vi "MagnetoGUI.vi"() -> ()   [LabVIEW 2016]
uses:
  controls/GUI Parameter.ctl
  controls/State.ctl
  controls/Data.ctl
panel:
  out "Tab Control":T1(tab)
  out "Aktueller Zustand":string
  in  "Taster Einstellungen":bool
  in  "Anz. Messpunkte Kommutierungskurve":i8=16 caption="Anz. Messpunkte\nKommutierungskurve" min=10 max=30 step=1
  out "Hystereseschleife und Kom.Kurve / Preview":cluster{dbl[], dbl[]}[](graph) caption="XY Graph"
  in  "Plot_Speichern":bool
  out "Status":bool
  in  "Start Button":bool
  in  "Maximieren":bool
  in  "GUI Parameter":T2={"Eisenquerschnitt [mm^2]"=30.0, "Wirksame Länge [cm]"=94.0, "Primärwindungszahl"=700.0, "Sekundärwindungszahl"=700.0, "Messwiderstand [Ohm]"=1.0, "Spannungsteilerverhaeltnis (1/x)"=1.0, "Probenbezeichnung"="", "Dichte des Eisens [g/cm^3]"=7.84, "magn. Flussdichte [T]"=2.0, "Frequenz [Hz]"=50.0, "Namen"="", "Gruppe"=""} {"Frequenz [Hz]" min=15.0 max=15000.0; "magn. Flussdichte [T]" min=0.001 max=5.0 step=0.05; "Dichte des Eisens [g/cm^3]" min=1.0 max=50.0 step=0.01; "Spannungsteilerverhaeltnis (1/x)" step=0.05; "Sekundärwindungszahl" min=1.0 max=1500.0; "Primärwindungszahl" min=1.0 max=1500.0; "Wirksame Länge [cm]" min=1.0 max=1000.0; "Eisenquerschnitt [mm^2]" min=1.0 max=10000.0}
  in  "Kommutierungskurve messen?":bool caption="Kommutierungskurve\nMessen?"
  in  "Maximal zulässiger Strom [A]":dbl=3.0 min=0.0 max=5.0 step=0.05
  in  "Minimale Spannung [V]":dbl=0.02 min=0.0 max=10.0
  in  "Maximale Spannung [V]":dbl=10.0 min=0.0 max=10.0
  out "Faktor2":dbl
  out "Faktor1":dbl
  out "TP":dbl caption="Theoretische Primärwindungszahl"
  in  "Taster Hauptansicht":bool
  in  "VISA Name Oszilloscope":refnum<visa-resource-name>="USB0::0x0957::0x179B::MY54313507::INSTR"
  in  "VISA Name Frequenzgen.":refnum<visa-resource-name>="USB0::0x0957::0x0407::MY44043889::INSTR"
  in  "Anzahl der Oszi-Messpunkte":i32=2000 min=2000 max=2000 step=1
  out "Bmax [T]":dbl
  out "Hmax [A/m]":dbl
  out "Koerzitivfeldstärke [A/m]":dbl caption="Koerzitiv-\nfeldstärke [A/m]"
  out "Remanenz [T]":dbl
  in  "Excel Export":bool
  out "Gruppe":string
  out "Namen":string
  out "Frequenz [Hz]":dbl
  out "magn. Flussdichte [T]":dbl
  out "Dichte des Eisens [g/cm^3]":dbl
  out "Probenbezeichnung":string
  out "Spannungsteilerverhältnis (1/x)":dbl
  out "Messwiderstand [Ohm]":dbl
  out "Sekundärwindungszahl":dbl
  out "Primärwindungszahl":dbl
  out "Wirksame Länge [cm]":dbl
  out "Eisenquerschnitt [mm^2]":dbl
  in  "Minimieren":bool
  in  "Ansicht_Speichern":bool
  out "Hystereseschleife und Kom.Kurve":cluster{dbl[], dbl[]}[](graph) caption="XY Graph"
  in  "Plot_Speichern 2":bool
  out "Datum/Uhrzeit":timestamp format="%<%H:%M\n%d/%m/%y>T"
  out "Hystereseverluste [W]":dbl
  # "Meldung merkerstromüberwachung"
  # "Meldung Frequenzgen im Spannungslimit"
  # "Laborversuch: Magnetische Eigenschaften"
  # "Laborversuch: Magnetische Eigenschaften"
  # "Oszilloskop Messpunkte"
  # "System Setup"
  # "Frequenzgenerator"
  # "Strombegrenzung"
  # "Anzeige der berechneten Größen"
  # "Laborversuch: Magnetische Eigenschaften"
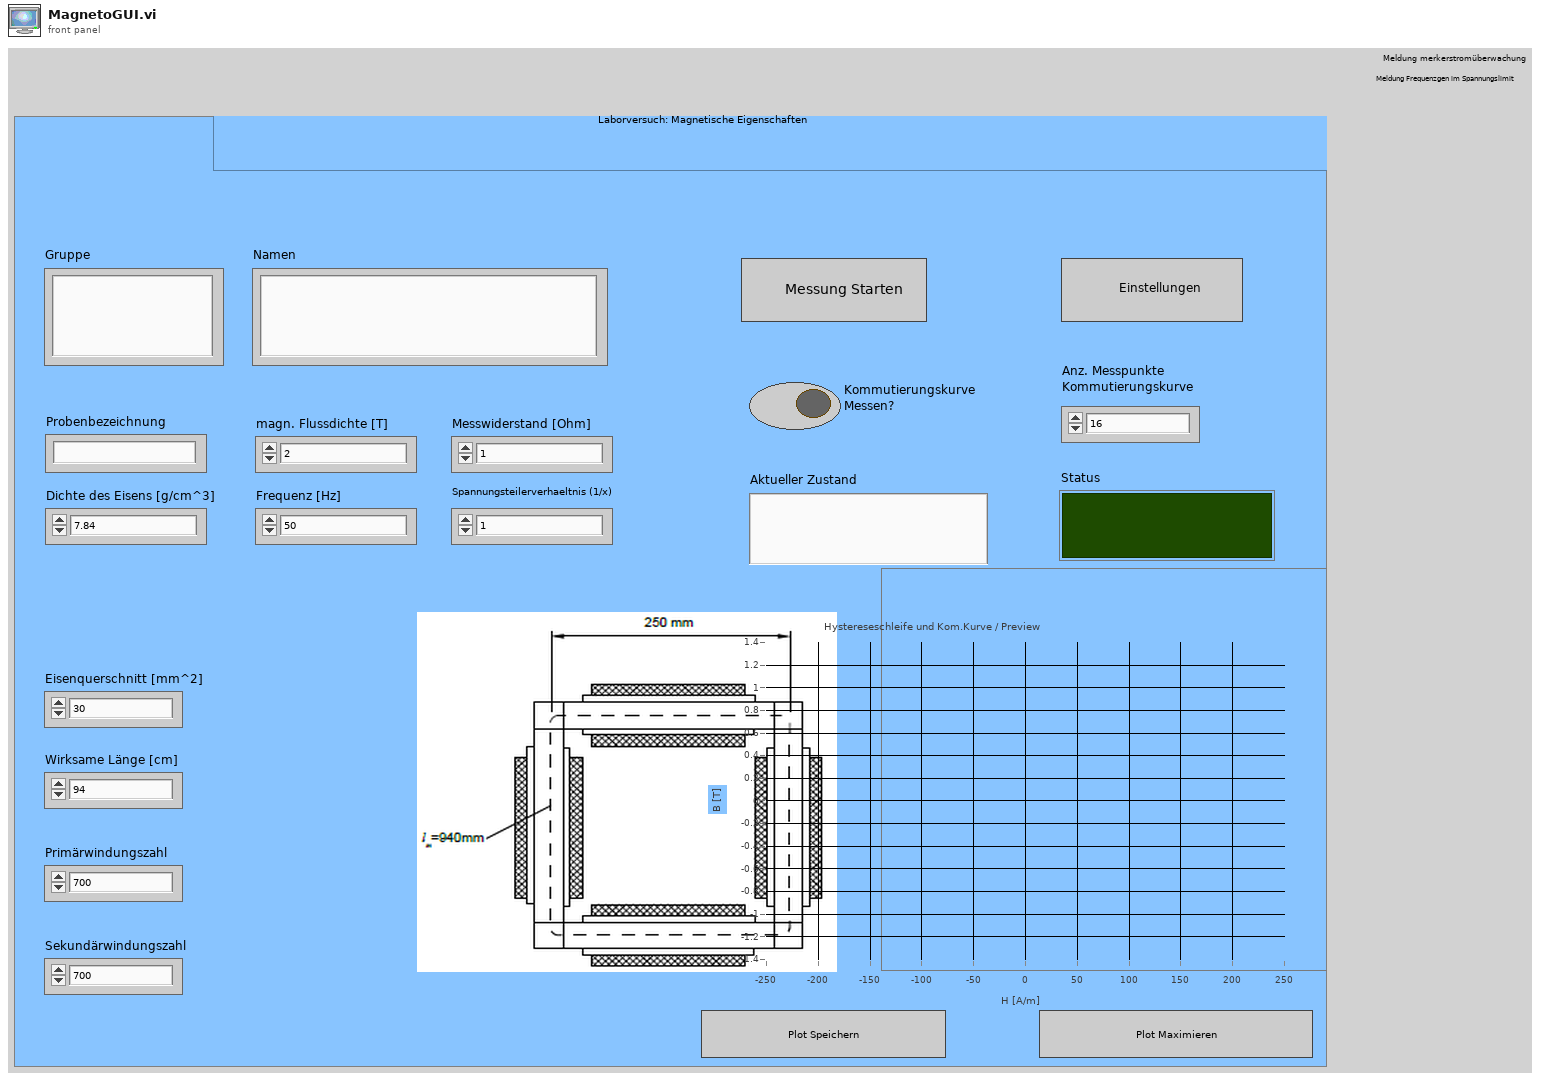
[diagram p1: front panel]
types:
  T1 = enum32{"Hauptansicht", "Optionen", "Plotansicht"}
  T2 = typedef "GUI Parameter.ctl" = cluster{"Eisenquerschnitt [mm^2]":dbl, "Wirksame Länge [cm]":dbl, "Primärwindungszahl":dbl, "Sekundärwindungszahl":dbl, "Messwiderstand [Ohm]":dbl, "Spannungsteilerverhaeltnis (1/x)":dbl, "Probenbezeichnung":string, "Dichte des Eisens [g/cm^3]":dbl, "magn. Flussdichte [T]":dbl, "Frequenz [Hz]":dbl, "Namen":string, "Gruppe":string}
  T3 = typedef "Data.ctl" = cluster{"GUI Einstellungen":cluster{"Maximale Spannung FG":dbl, "Faktor1":dbl, "Faktor2":dbl, "Theoretische Primärwindungszahl":dbl, "Anzahl der Messpunkte":i32, "VISA Name Oszilloscope":refnum<visa-resource-name>, "VISA Name Frequenzgenerator":refnum<visa-resource-name>, "Minimale Spannung FG":dbl, "Pfad für Messwerte und Plots":path, "Maximal Strom [A] ":dbl}, "GUI Daten":cluster{"Eisenquerschnitt [mm^2]":dbl, "Wirksame Länge [cm]":dbl, "Primärwindungszahl":dbl, "Sekundärwindungszahl":dbl, "Messwiderstand [Ohm]":dbl, "Spannungsteilerverhaeltnis (1/x)":dbl, "Probenbezeichnung":string, "Dichte des Eisens [g/cm^3]":dbl, "magn. Flussdichte [T]":dbl, "Frequenz [Hz]":dbl, "Namen":string, "Gruppe":string}, "Messung Hystereseschleife":cluster{"Hystereseverluste":dbl, "B - Hysterese Array":dbl[], "H - Hysterese Array":dbl[], "Hmax":dbl, "Bmax":dbl, "Remanenz":dbl, "Koerzitivfeldstärke":dbl}, "Messung Neukurve":cluster{"Neukurve Messen?":bool, "Anzahl Messpunkte Neukurve":i8, "B - Neukurve Array":dbl[], "H - Neukurve Array":dbl[]}, "Globale Variablen":cluster{"Max Spannung\nerreicht?":bool, "Min Spannung\nerreicht?":bool, "Keine Neu- oder\nKommutierungskurvenmessung\nmoeglich":bool, "bmax1":dbl, "bmin1":dbl, "bmax2":dbl, "bmin2":dbl, "Spannungsabweichung":dbl, "Tatsächliche Flussdichte":dbl, "Tatsächliche \nAnzahl Punkte":dbl, "hmax1":dbl, "hmin1":dbl, "hmax2":dbl, " Strombegrenzung aktiv?":bool, "Abbruch Messung":bool}}
  T4 = typedef "State.ctl" = enum16{"Initialisieren", "Warten auf Event", "Starten der Messung", "Initialisieren Hardware", "Flussdichte Einstellen", "Chk Flussdichte Anpassung", "Messung Hystereseschleife", "Entmagnetisieren", "Messung Kommutierungskurve", "Entmagnetisieren 2", "Ausgabe Diagramm", "Ende", "Plot aufnehmen", "Ansicht speichern", "Excel Export"}
  T5 = cluster{"Maximale Spannung FG":dbl, "Faktor1":dbl, "Faktor2":dbl, "Theoretische Primärwindungszahl":dbl, "Anzahl der Messpunkte":i32, "VISA Name Oszilloscope":refnum<visa-resource-name>, "VISA Name Frequenzgenerator":refnum<visa-resource-name>, "Minimale Spannung FG":dbl, "Pfad für Messwerte und Plots":path, "Maximal Strom [A] ":dbl}
  T6 = cluster{"Eisenquerschnitt [mm^2]":dbl, "Wirksame Länge [cm]":dbl, "Primärwindungszahl":dbl, "Sekundärwindungszahl":dbl, "Messwiderstand [Ohm]":dbl, "Spannungsteilerverhaeltnis (1/x)":dbl, "Probenbezeichnung":string, "Dichte des Eisens [g/cm^3]":dbl, "magn. Flussdichte [T]":dbl, "Frequenz [Hz]":dbl, "Namen":string, "Gruppe":string}
  T7 = cluster{"Max Spannung\nerreicht?":bool, "Min Spannung\nerreicht?":bool, "Keine Neu- oder\nKommutierungskurvenmessung\nmoeglich":bool, "bmax1":dbl, "bmin1":dbl, "bmax2":dbl, "bmin2":dbl, "Spannungsabweichung":dbl, "Tatsächliche Flussdichte":dbl, "Tatsächliche \nAnzahl Punkte":dbl, "hmax1":dbl, "hmin1":dbl, "hmax2":dbl, " Strombegrenzung aktiv?":bool, "Abbruch Messung":bool}
  T8 = cluster{"Max Spannung\nerreicht?":bool, "Min Spannung\nerreicht?":bool, "Keine Neu- oder\nKommutierungskurvenmessung\nmoeglich":bool, "bmax1":dbl, "bmin1":dbl, "bmax2":dbl, "bmin2":dbl, "Spannungsabweichung":dbl, "Tatsächliche Flussdichte":dbl, "Tatsächliche \nAnzahl Punkte":dbl, "hmax1":dbl, "hmin1":dbl, "hmax2":dbl, " Stromueberwachung aktiv?":bool, "Abbruch Messung":bool}
  T9 = cluster{"Hystereseverluste":dbl, "B - Hysterese Array":dbl[], "H - Hysterese Array":dbl[], "Hmax":dbl, "Bmax":dbl, "Remanenz":dbl, "Koerzitivfeldstärke":dbl}
  T10 = cluster{"H - Hysterese Array":dbl[], "B - Hysterese Array":dbl[]}
  T11 = cluster{"H - Neukurve Array":dbl[], "B - Neukurve Array":dbl[]}
  T12 = cluster{"H - Neukurve Array":dbl[], "B - Neukurve Array":dbl[]}[]
  T13 = typedef "imagedata.ctl" = cluster{"image type":i32, "image depth":i32, "image":u8[], "mask":u8[], "colors":u32[], "Rectangle":cluster{"left":i16, "top":i16, "right":i16, "bottom":i16}}
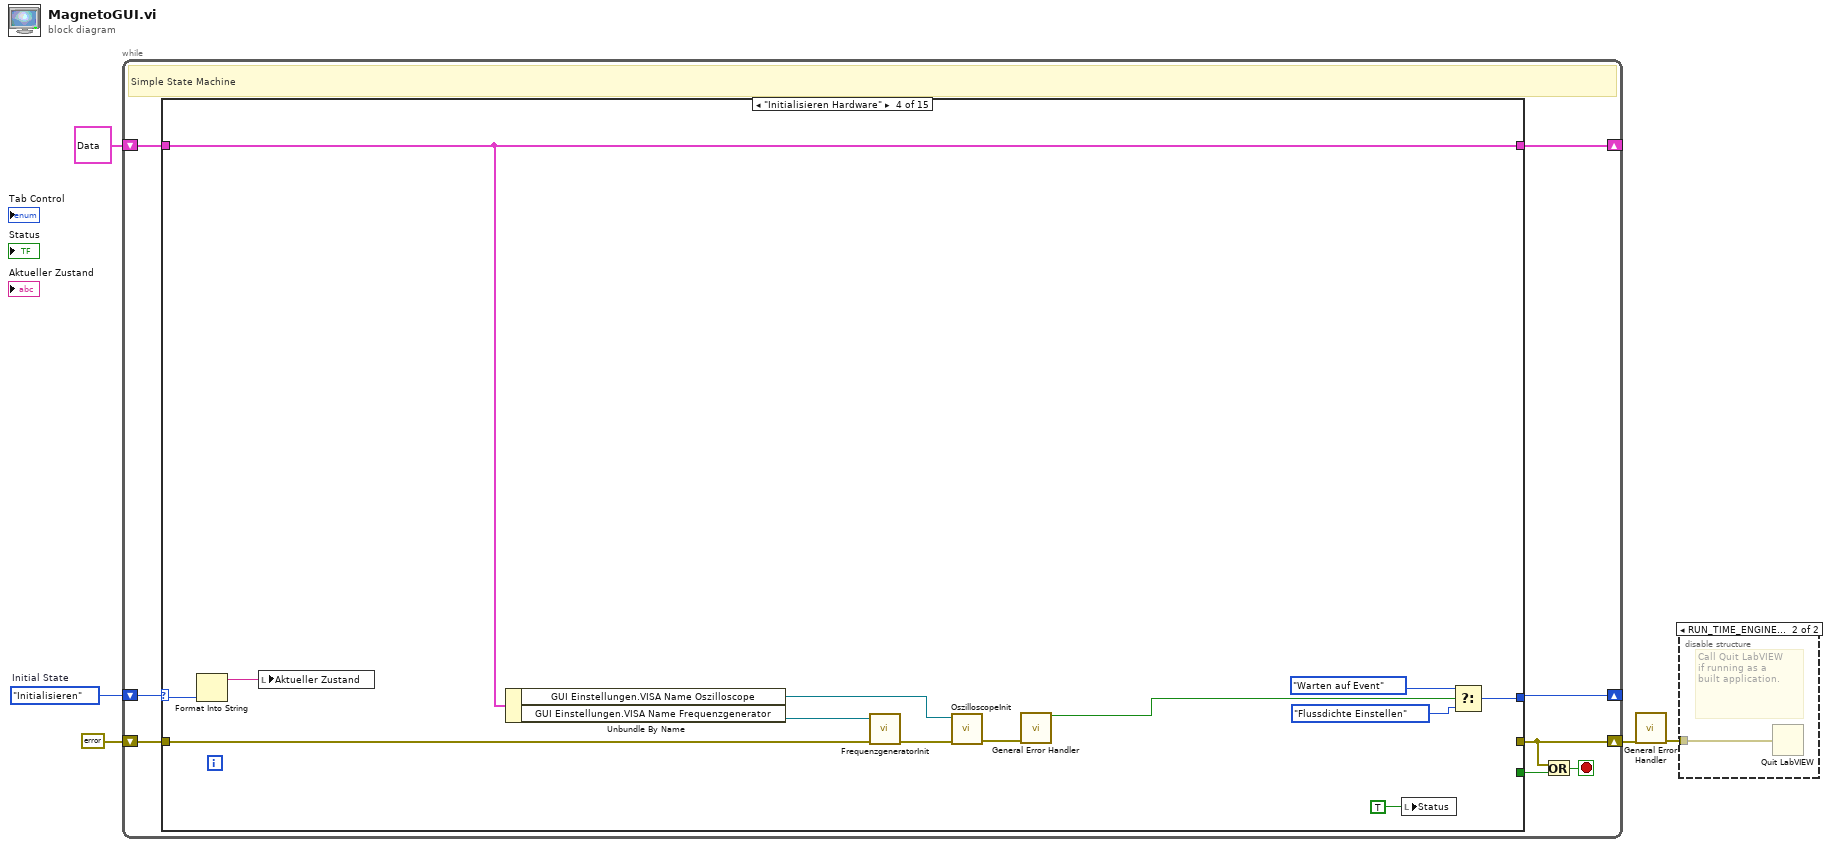
[diagram p0: block diagram]
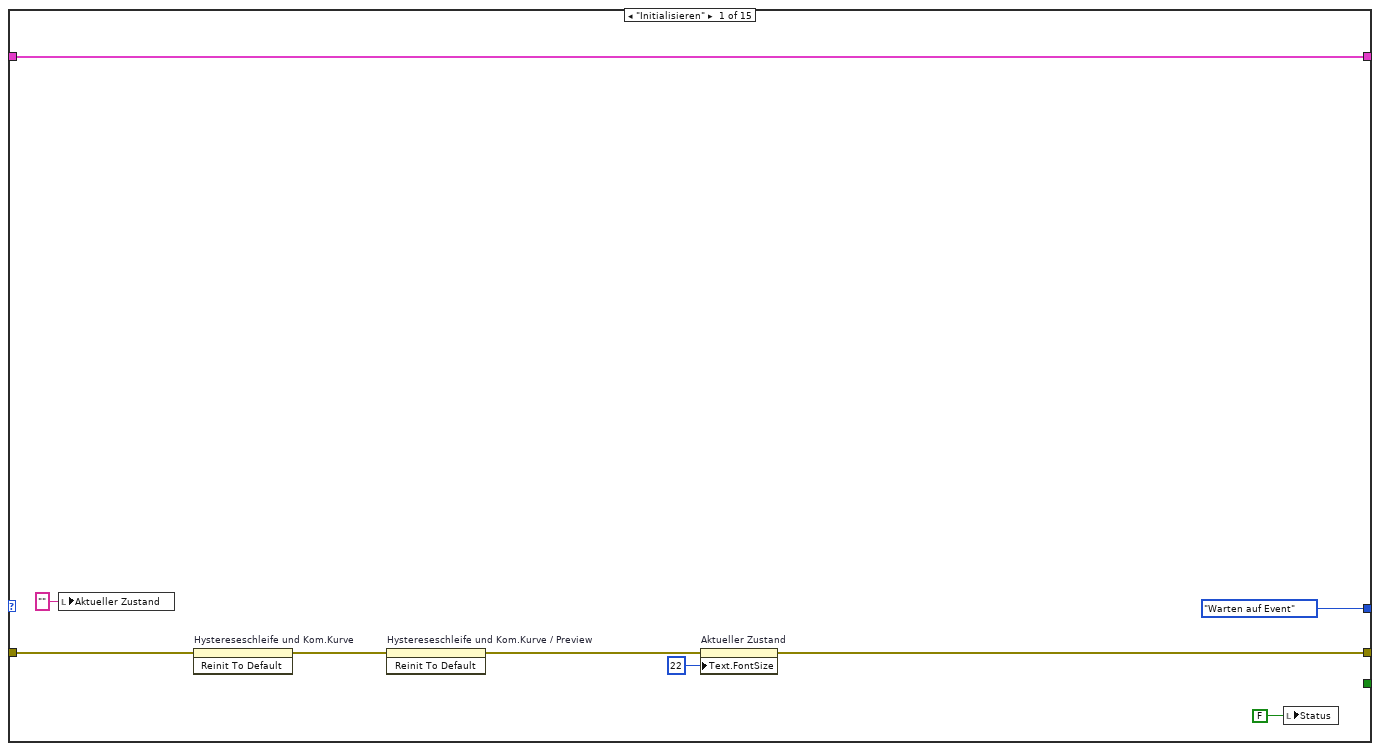
[diagram p3: hidden frame]
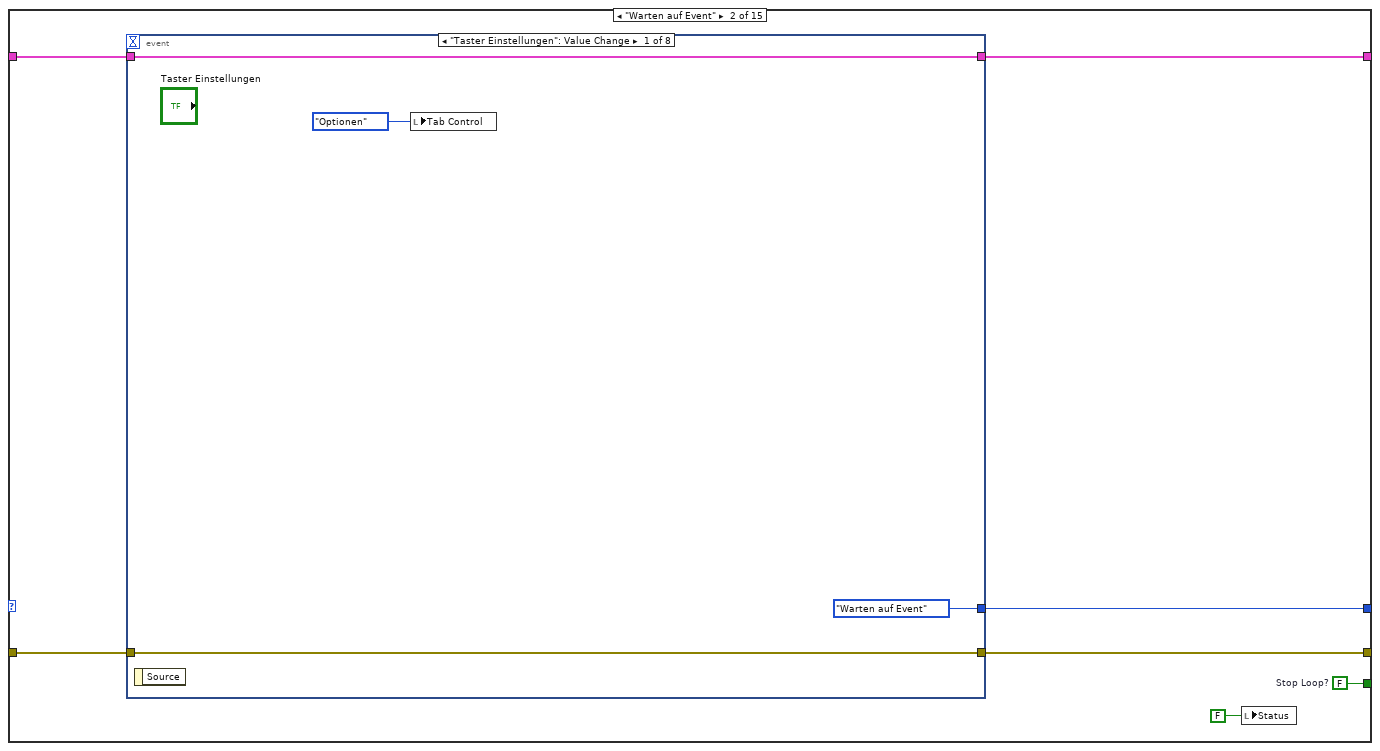
[diagram p4: hidden frame]
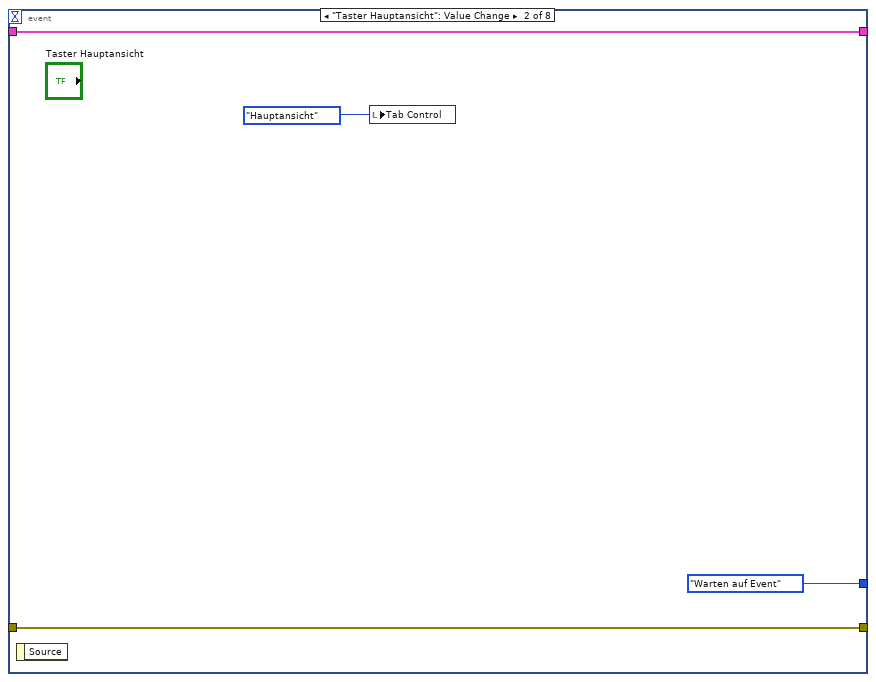
[diagram p5: hidden frame]
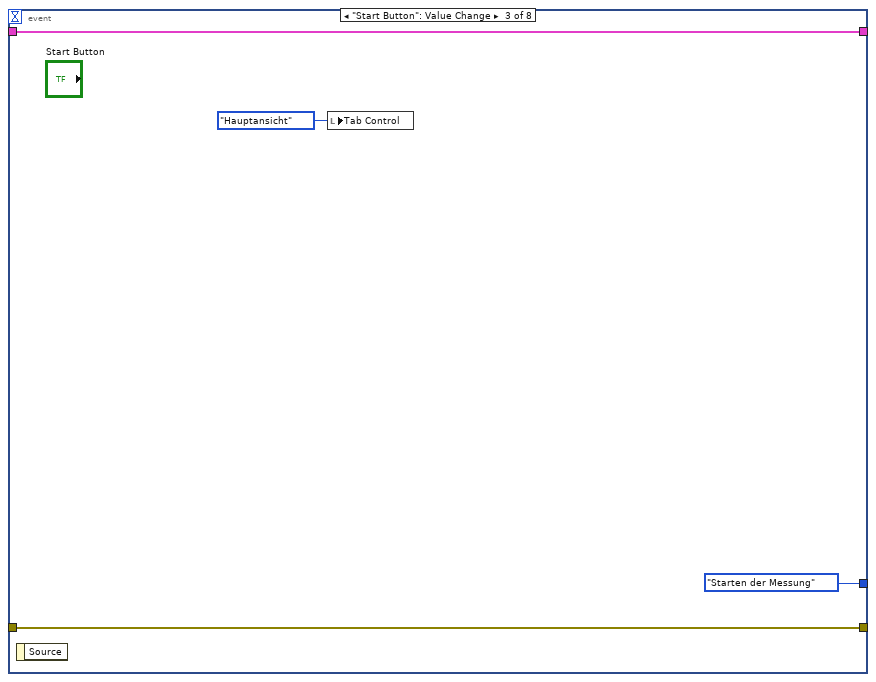
[diagram p6: hidden frame]
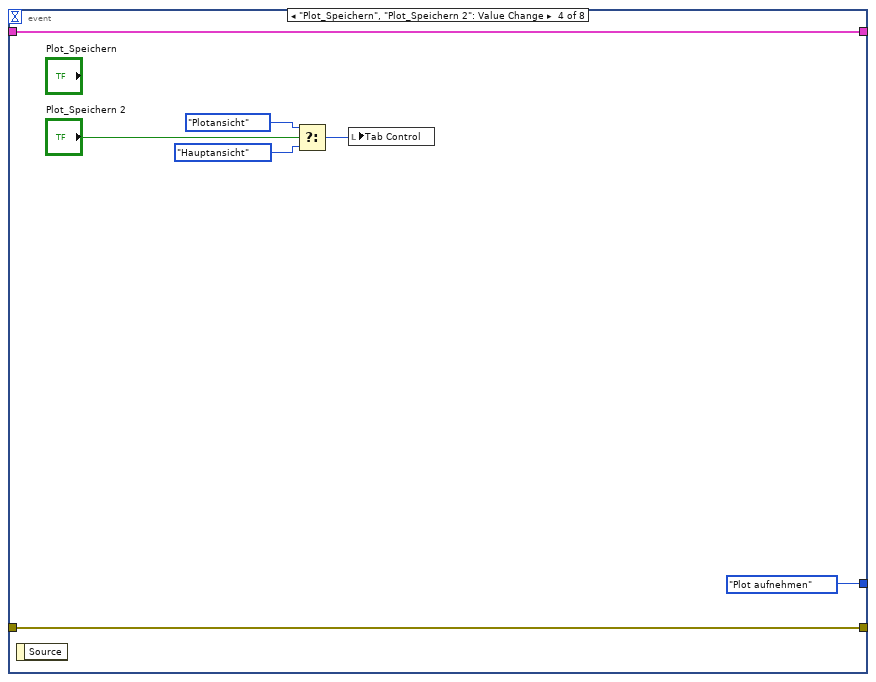
[diagram p7: hidden frame]
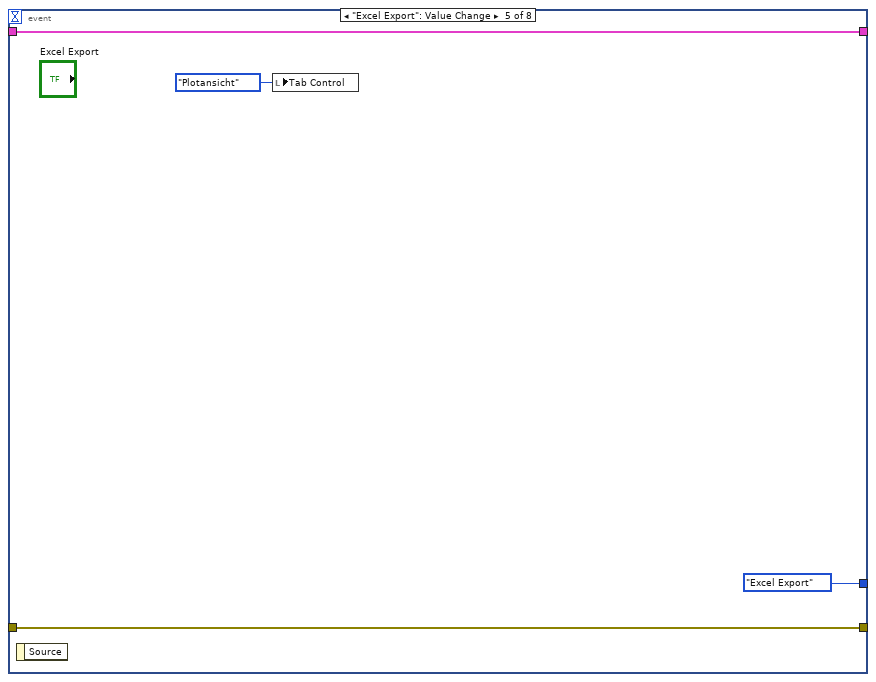
[diagram p8: hidden frame]
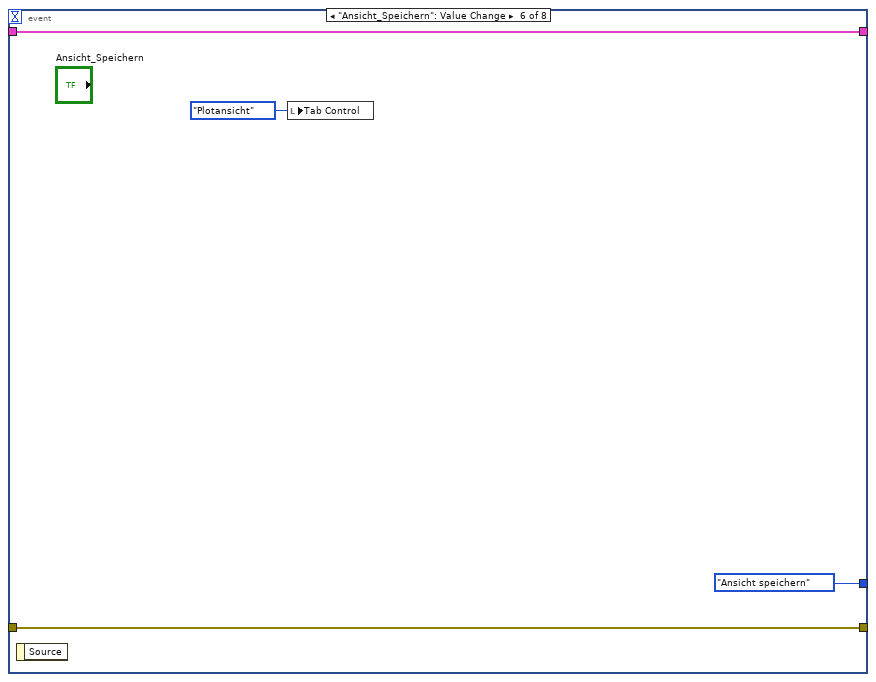
[diagram p9: hidden frame]
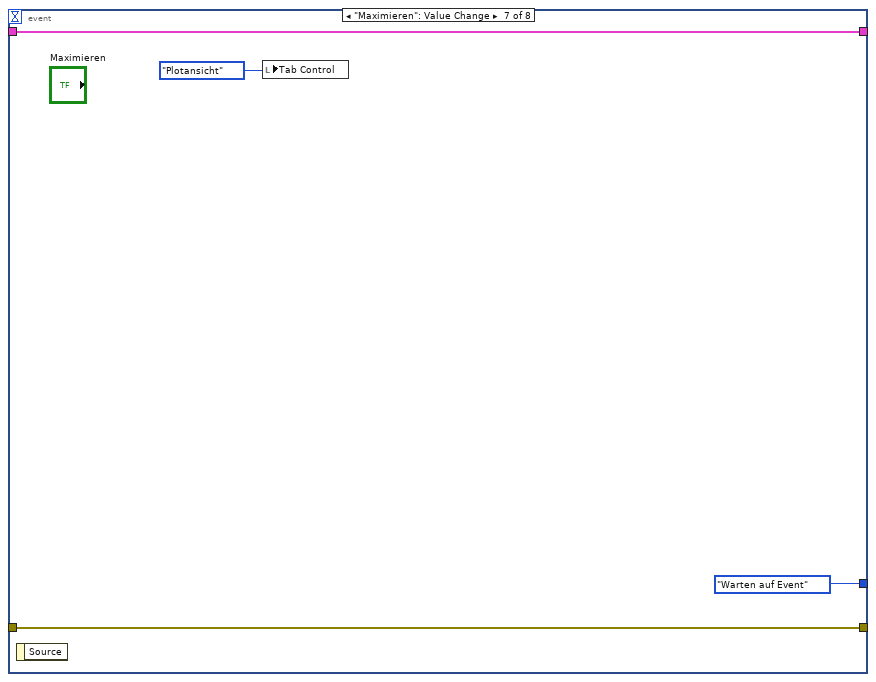
[diagram p10: hidden frame]
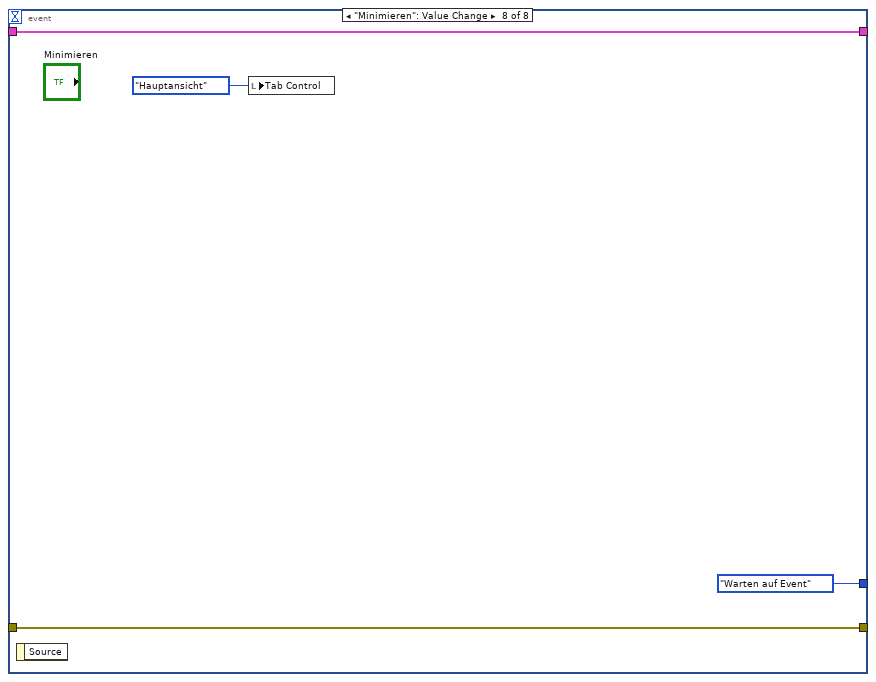
[diagram p11: hidden frame]
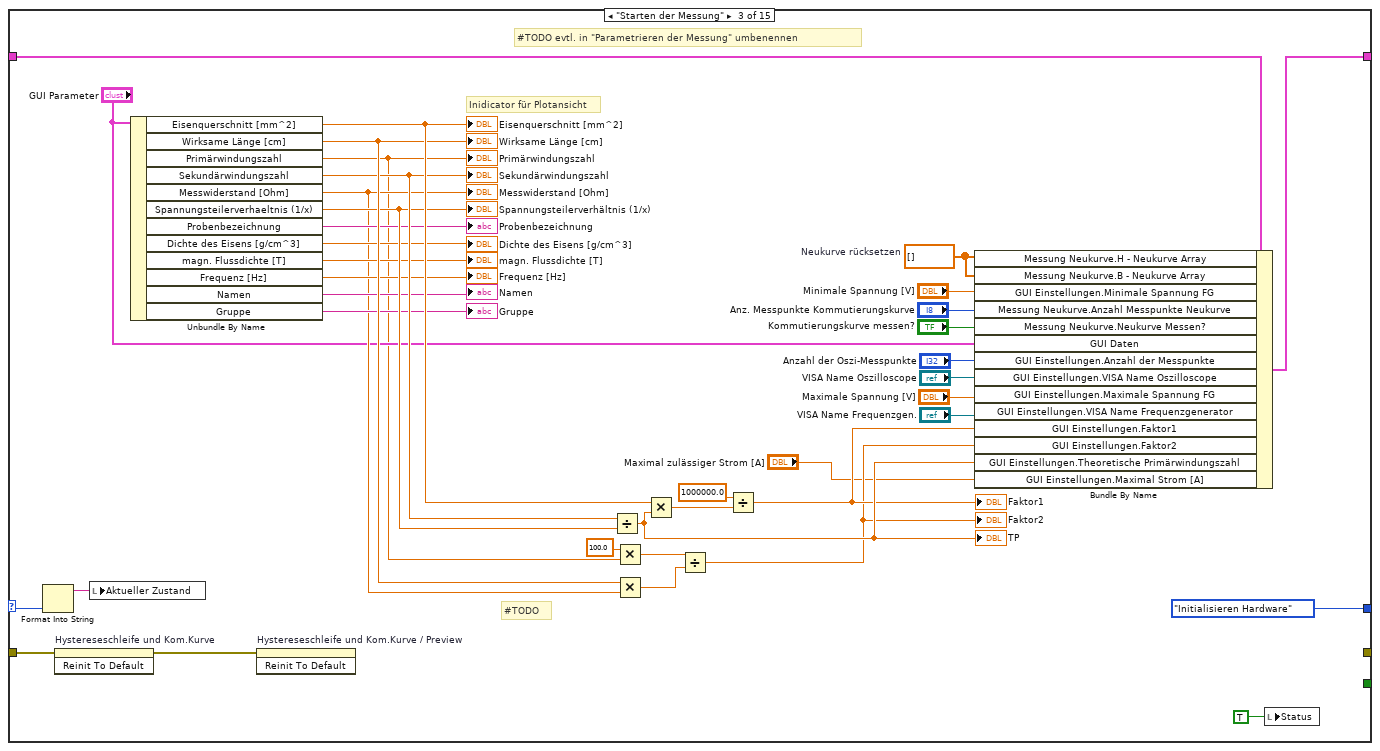
[diagram p12: hidden frame]
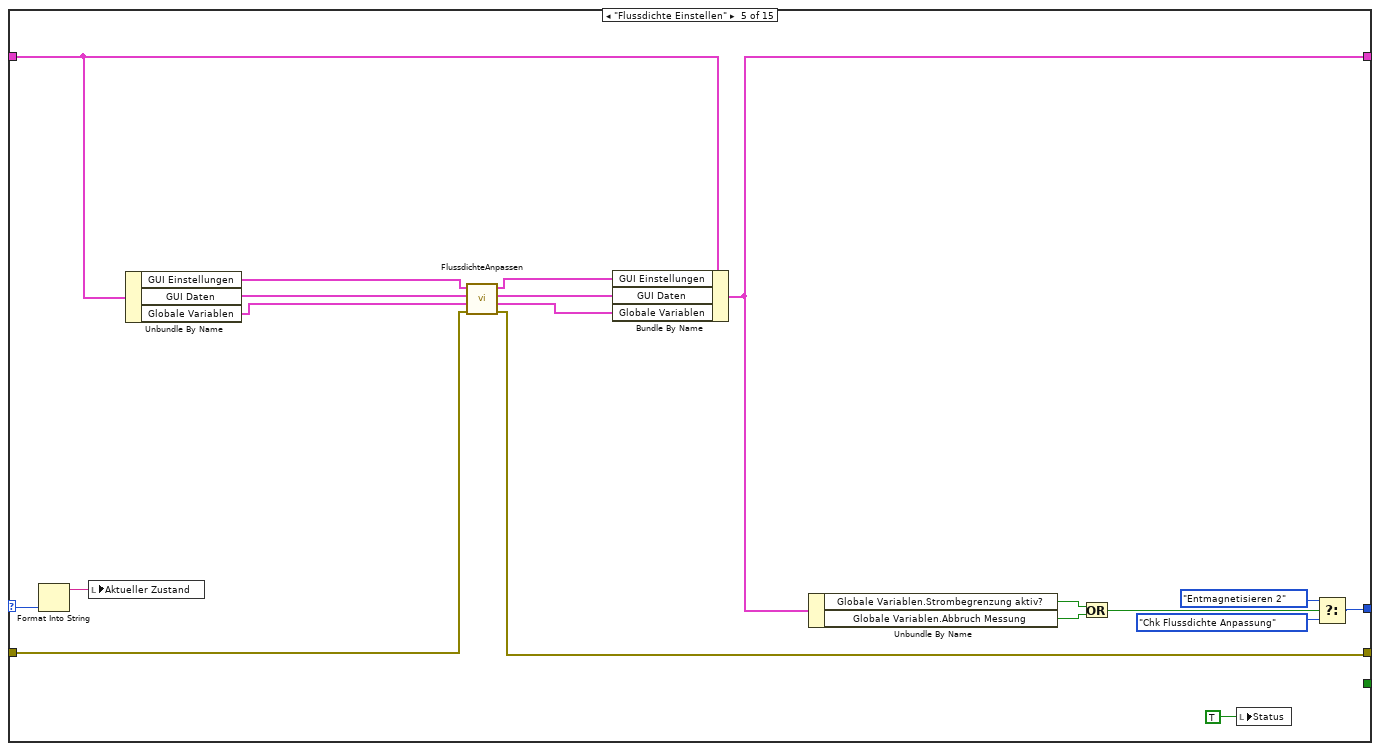
[diagram p13: hidden frame]
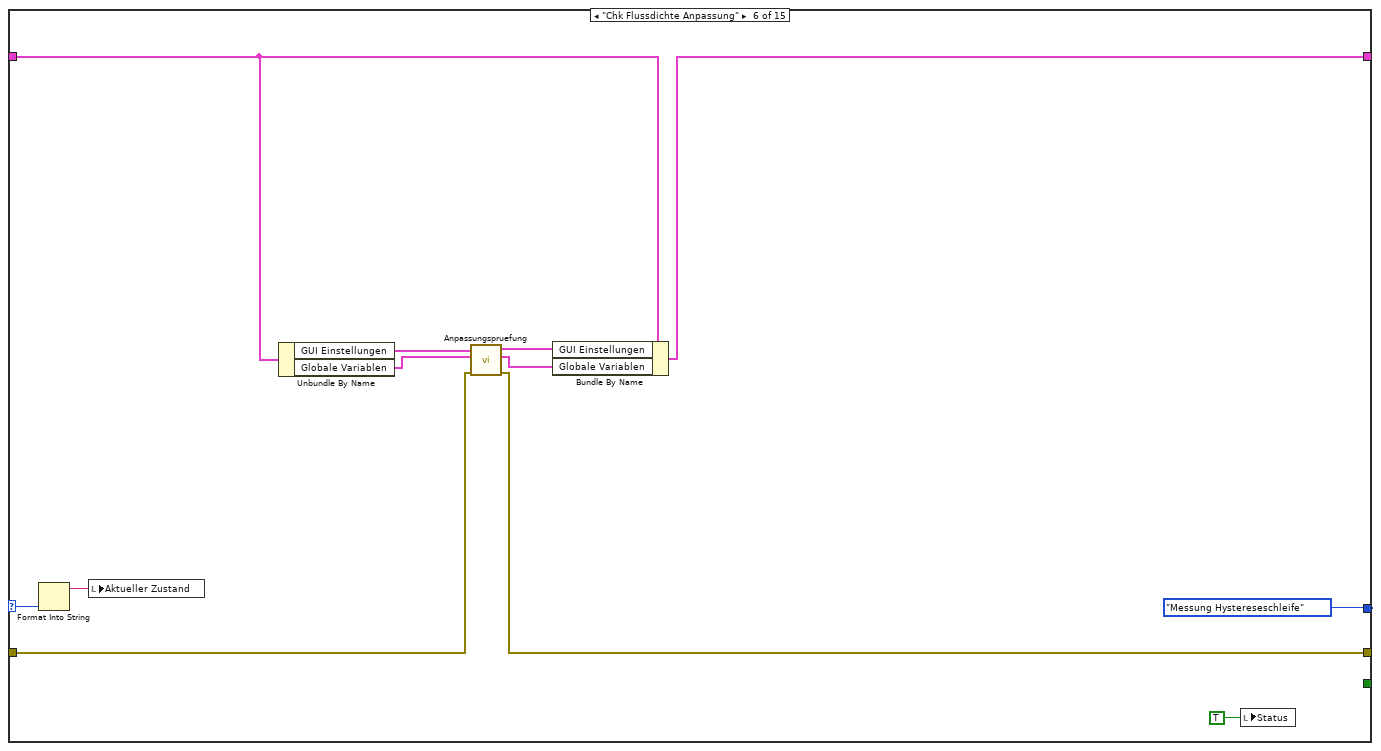
[diagram p14: hidden frame]
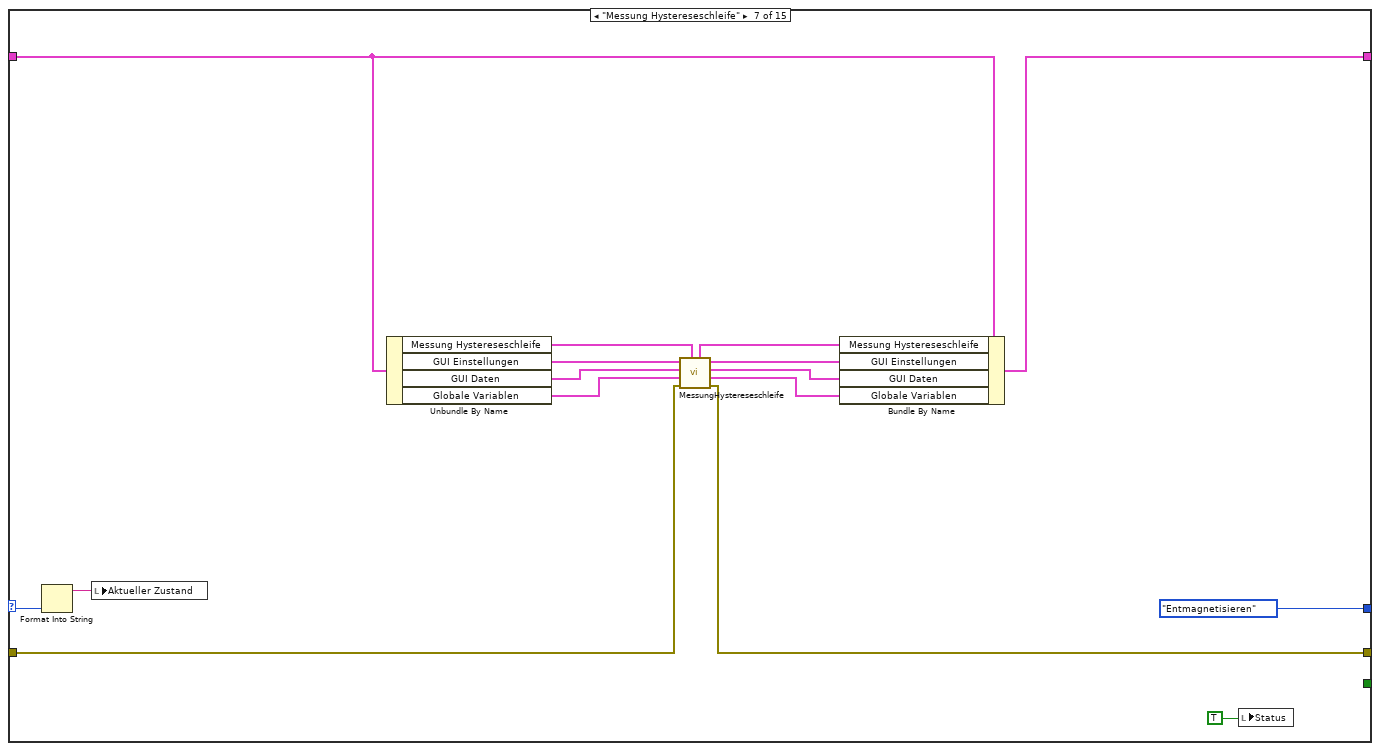
[diagram p15: hidden frame]
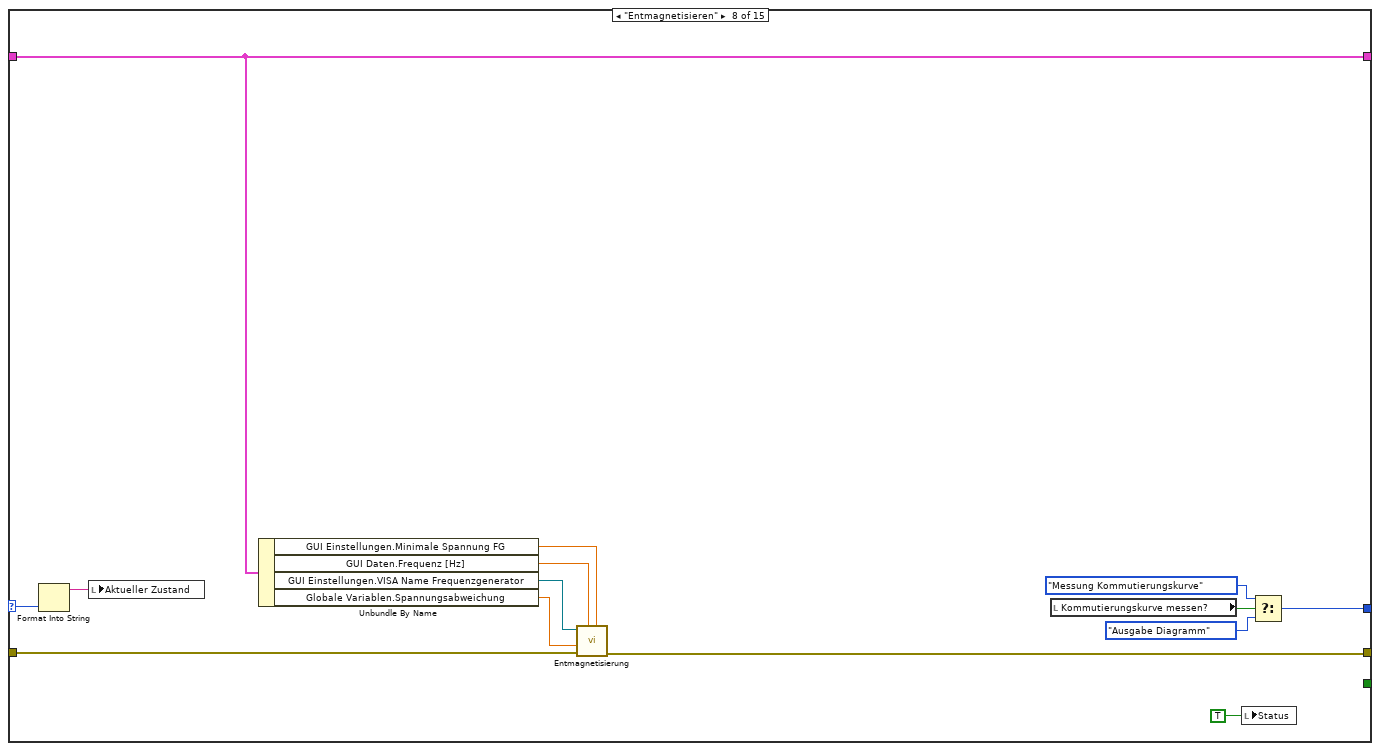
[diagram p16: hidden frame]
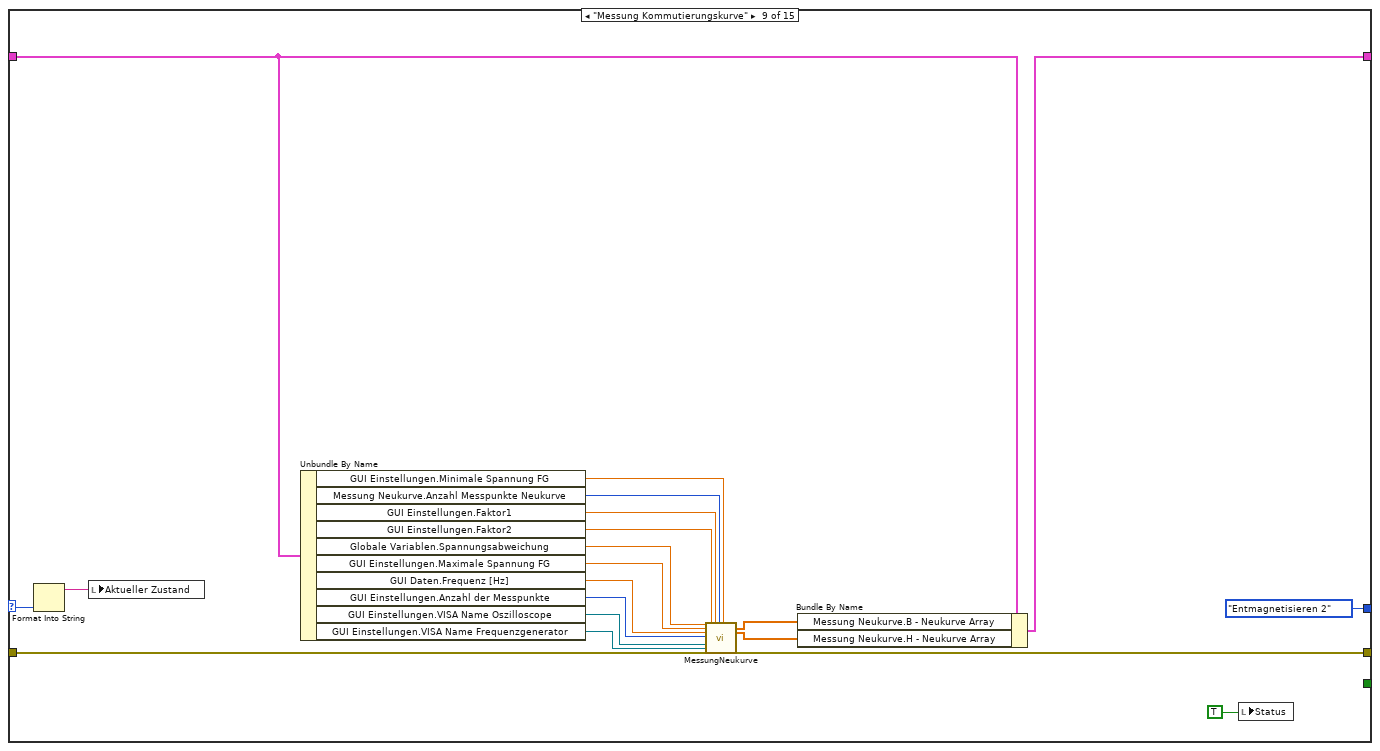
[diagram p17: hidden frame]
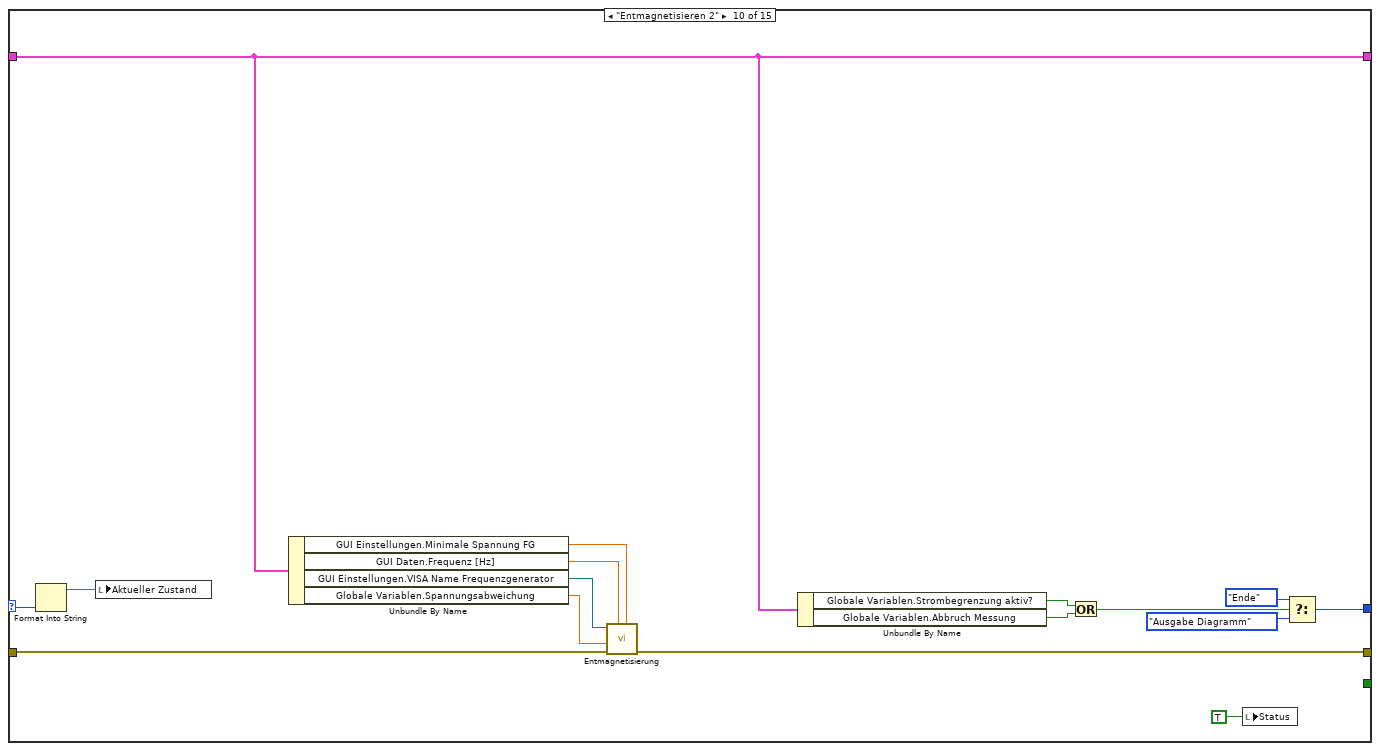
[diagram p18: hidden frame]
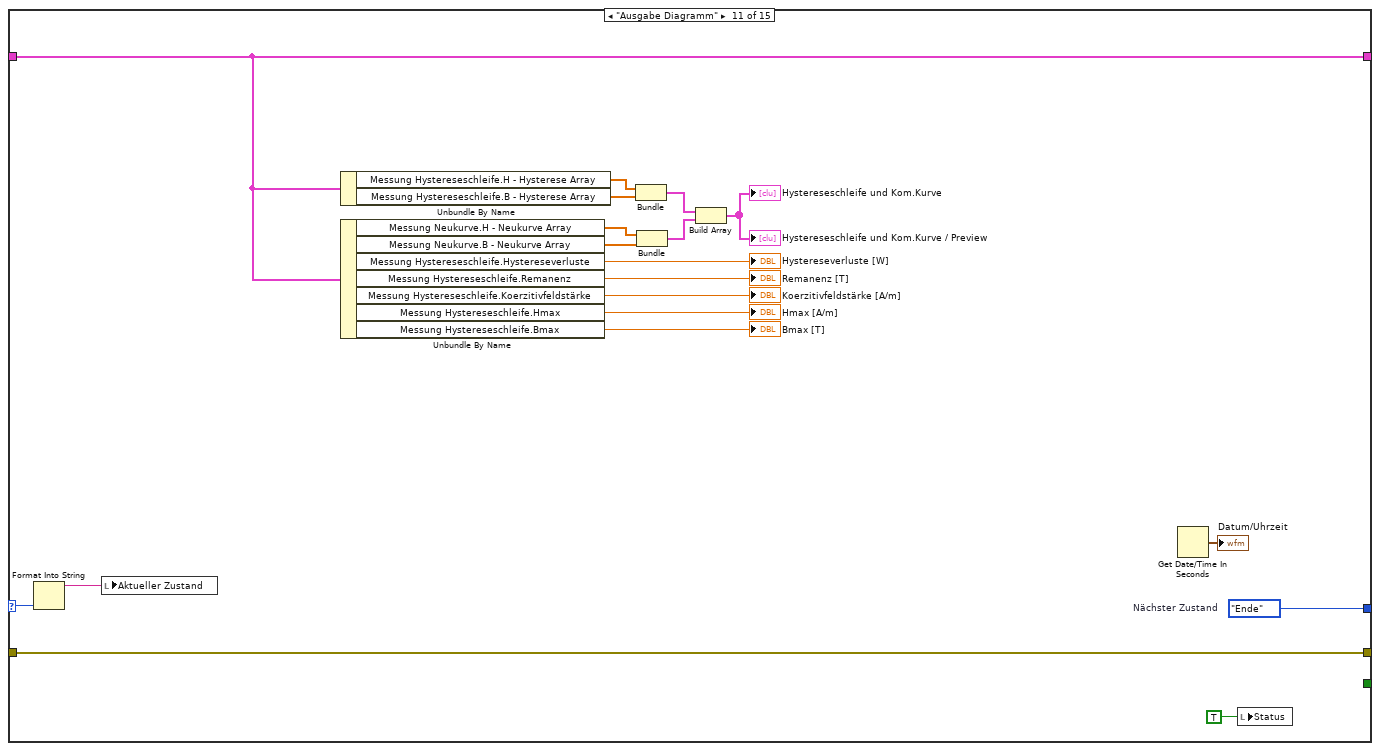
[diagram p19: hidden frame]
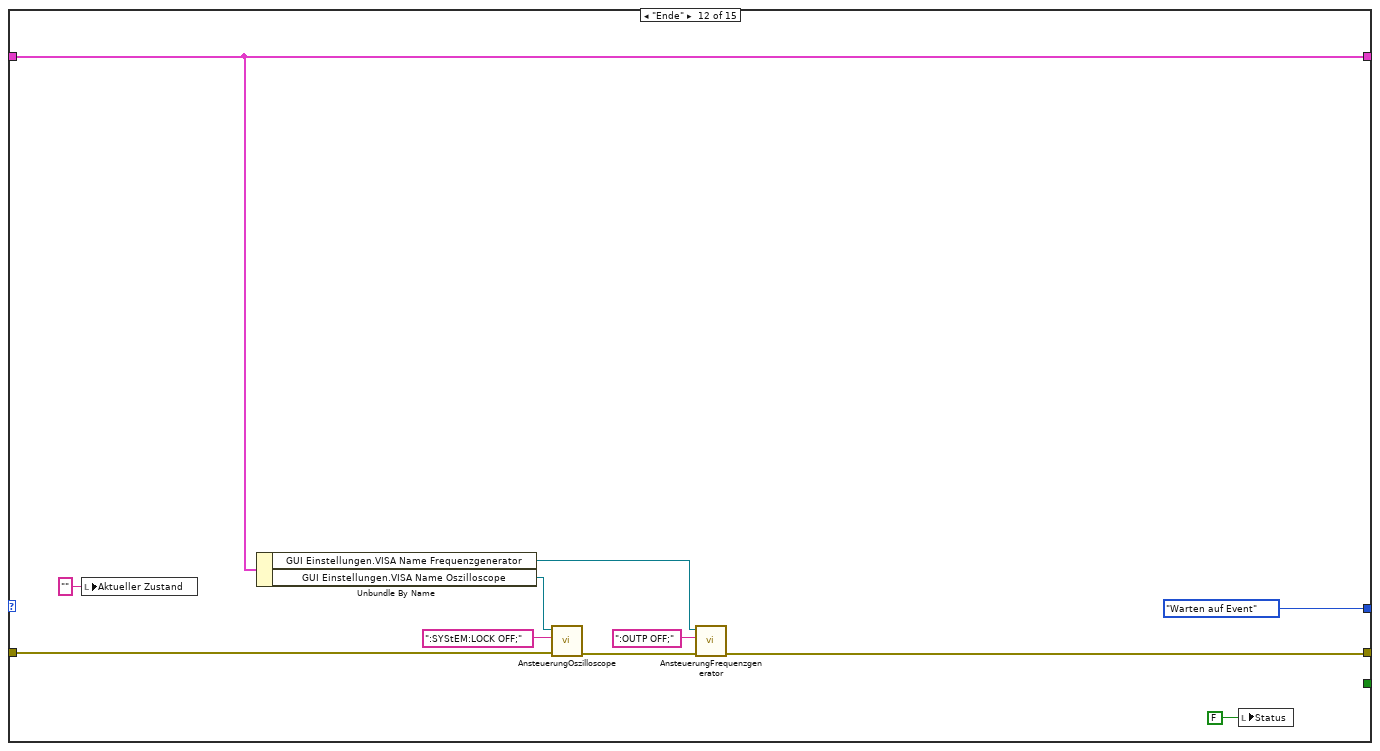
[diagram p20: hidden frame]
diagram:
  w1 = State."Initialisieren"  # Initial State
  n1 = while {
    shift-right: [w12] -> _
    shift-left: w1 -> [w13]
    shift-right: [w10] -> _
    shift-left: T3 {"GUI Einstellungen"={"Maximale Spannung FG"=0.0, "Faktor1"=0.0, "Faktor2"=0.0, "Theoretische Primärwindungszahl"=0.0, "Anzahl der Messpunkte"=0, "VISA Name Oszilloscope"="", "VISA Name Frequenzgenerator"="", "Minimale Spannung FG"=0.0, "Pfad für Messwerte und Plots"=path "", "Maximal Strom [A] "=0.5}, "GUI Daten"={"Eisenquerschnitt [mm^2]"=0.0, "Wirksame Länge [cm]"=0.0, "Primärwindungszahl"=0.0, "Sekundärwindungszahl"=0.0, "Messwiderstand [Ohm]"=0.0, "Spannungsteilerverhaeltnis (1/x)"=0.0, "Probenbezeichnung"="", "Dichte des Eisens [g/cm^3]"=0.0, "magn. Flussdichte [T]"=0.0, "Frequenz [Hz]"=0.0, "Namen"="", "Gruppe"=""}, "Messung Hystereseschleife"={"Hystereseverluste"=0.0, "B - Hysterese Array"=[0.0, 0.0], "H - Hysterese Array"=[0.0, 0.0], "Hmax"=0.0, "Bmax"=0.0, "Remanenz"=0.0, "Koerzitivfeldstärke"=0.0}, "Messung Neukurve"={"Neukurve Messen?"=FALSE, "Anzahl Messpunkte Neukurve"=16, "B - Neukurve Array"=[], "H - Neukurve Array"=[]}, "Globale Variablen"={"Max Spannung\nerreicht?"=FALSE, "Min Spannung\nerreicht?"=FALSE, "Keine Neu- oder\nKommutierungskurvenmessung\nmoeglich"=FALSE, "bmax1"=0.0, "bmin1"=0.0, "bmax2"=0.0, "bmin2"=0.0, "Spannungsabweichung"=0.0, "Tatsächliche Flussdichte"=0.0, "Tatsächliche \nAnzahl Punkte"=0.0, "hmax1"=0.0, "hmin1"=0.0, "hmax2"=0.0, " Strombegrenzung aktiv?"=FALSE, "Abbruch Messung"=FALSE}} ("Data") -> [w11]
    shift-right: [w7] -> w3
    shift-left: errorcluster {"status"=FALSE, "code"=0, "source"=""} ("error constant") -> [w9]
    stop <- w8 stop-if-true
    # "Simple State Machine"
    n2 = case shown="\"Initialisieren Hardware\"" w13 {
      selector: w13 -> [_ _ w68 w108 w129 w141 w155 w164 w178 w205 w220 _ _ _ _]
      tunnel: [State."Warten auf Event" ("Next State") w29 State."Initialisieren Hardware" ("Next State") w106 w117 State."Messung Hystereseschleife" ("Next  State") State."Entmagnetisieren" ("(Value Not Used)") w169 State."Entmagnetisieren 2" ("Initial State") w201 w230 State."Warten auf Event" ("Next  State") State."Warten auf Event" ("Next  State") State."Warten auf Event" ("Next  State") State."Warten auf Event" ("Next  State")] -> w12
      tunnel: w11 -> [w21 w28 w84 w115 w127 w146 w159 w176 w186 w198 w225 w241 w249 w256 w262]
      tunnel: [w21 w27 w85 w115 w116 w140 w162 w176 w190 w198 w225 w241 w249 w256 w262] -> w10
      tunnel: w9 -> [w20 w26 w102 w114 w133 w144 w158 w175 w196 w209 w229 w242 w247 w252 w260]
      tunnel: [w14 w25 _ _ w128 w145 w160 w167 w195 w208 w229 w232 _ _ _] -> w7
      tunnel: [_ w23 _ _ _ _ _ _ _ _ _ _ _ _ _] -> w6
      frame "Initialisieren" {
        n3 = local write "Aktueller Zustand"("" ("Aktueller Zustand")) -> ()
        n4 = invoke on="Hystereseschleife und Kom.Kurve" class="XYGraph (strikt)" method="Reinit To Default"(error in=w20) -> (error out=w19:errorcluster)  [unwired: 2 in, 2 out]
        n5 = invoke on="Hystereseschleife und Kom.Kurve / Preview" class="XYGraph (strikt)" method="Reinit To Default"(error in=w19) -> (error out=w17:errorcluster)  [unwired: 2 in, 2 out]
        n6 = property on="Aktueller Zustand" class="Str"(error in=w17, "Text.FontSize"=22) -> (error out=w14:errorcluster)  [unwired: 1 in, 1 out]
        n7 = local write "Status"(FALSE ("Status")) -> ()
      }
      frame "Warten auf Event" {
        w23 = FALSE  # Stop Loop?
        n8 = event shown="[0] \"Taster Einstellungen\": Value Change" {
          selector: _ -> [_ _ _ _ _ _ _ _]
          dyn-events: _ -> [_ _ _ _ _ _ _ _]
          timeout: _ -> [_ _ _ _ _ _ _ _]
          tunnel: [State."Warten auf Event" State."Warten auf Event" ("Next State") State."Starten der Messung" ("Next State") State."Plot aufnehmen" ("Next State") State."Excel Export" ("Next State") State."Ansicht speichern" ("Next State") State."Warten auf Event" ("Next State") State."Warten auf Event" ("Next State")] -> w29
          tunnel: w28 -> [w33 w37 w39 w48 w52 w56 w58 w64]
          tunnel: [w33 w37 w39 w48 w52 w56 w58 w64] -> w27
          tunnel: w26 -> [w32 w36 w40 w42 w49 w53 w59 w63]
          tunnel: [w32 w36 w40 w42 w49 w53 w59 w63] -> w25
          event "Taster Einstellungen": Value Change {
            n9 = event-data() -> ()  [unwired: 1 in, 1 out]
            n10 = local write "Tab Control"(T1."Optionen" ("Tab Control")) -> ()
          }
          event "Taster Hauptansicht": Value Change {
            n11 = event-data() -> ()  [unwired: 1 in, 1 out]
            n12 = local write "Tab Control"(T1."Hauptansicht" ("Tab Control")) -> ()
          }
          event "Start Button": Value Change {
            n13 = event-data() -> ()  [unwired: 1 in, 1 out]
            n14 = local write "Tab Control"(T1."Hauptansicht" ("Tab Control")) -> ()
          }
          event "Plot_Speichern", "Plot_Speichern 2": Value Change {
            n15 = event-data() -> ()  [unwired: 1 in, 1 out]
            n16 = Select(t=T1."Plotansicht" ("Tab Control"), s="Plot_Speichern 2", f=T1."Hauptansicht" ("Tab Control")) -> (s? t:f=w43:T1)
            n17 = local write "Tab Control"(w43) -> ()
          }
          event "Excel Export": Value Change {
            n18 = event-data() -> ()  [unwired: 1 in, 1 out]
            n19 = local write "Tab Control"(T1."Plotansicht" ("Tab Control")) -> ()
          }
          event "Ansicht_Speichern": Value Change {
            n20 = event-data() -> ()  [unwired: 1 in, 1 out]
            n21 = local write "Tab Control"(T1."Plotansicht" ("Tab Control")) -> ()
          }
          event "Maximieren": Value Change {
            n22 = event-data() -> ()  [unwired: 1 in, 1 out]
            n23 = local write "Tab Control"(T1."Plotansicht" ("Tab Control")) -> ()
          }
          event "Minimieren": Value Change {
            n24 = event-data() -> ()  [unwired: 1 in, 1 out]
            n25 = local write "Tab Control"(T1."Hauptansicht" ("Tab Control")) -> ()
          }
        }
        n26 = local write "Status"(FALSE ("Status")) -> ()
      }
      frame "Starten der Messung" {
        w66 = dbl[] []  # Neukurve rücksetzen
        # "#TODO evtl. in \"Parametrieren der Messung\" umbenennen"
        # "#TODO"
        # "Inidicator für Plotansicht"
        n27 = Format Into String(w68) -> (resulting string=w70:string)  [unwired: 3 in, 1 out]
        n28 = invoke on="Hystereseschleife und Kom.Kurve" class="XYGraph (strict)" method="Reinit To Default"(error in=w102) -> (error out=w101:errorcluster)  [unwired: 2 in, 2 out]
        n29 = local write "Aktueller Zustand"(w70) -> ()
        n30 = Unbundle By Name("GUI Parameter") -> ("Eisenquerschnitt [mm^2]"=w95:dbl, "Wirksame Länge [cm]"=w94:dbl, "Primärwindungszahl"=w65:dbl, "Sekundärwindungszahl"=w93:dbl, "Messwiderstand [Ohm]"=w83:dbl, "Spannungsteilerverhaeltnis (1/x)"=w92:dbl, "Probenbezeichnung"=→"Probenbezeichnung":string, "Dichte des Eisens [g/cm^3]"=→"Dichte des Eisens [g/cm^3]":dbl, "magn. Flussdichte [T]"=→"magn. Flussdichte [T]":dbl, "Frequenz [Hz]"=→"Frequenz [Hz]":dbl, "Namen"=→"Namen":string, "Gruppe"=→"Gruppe":string)
        "Eisenquerschnitt [mm^2]" <- w95
        "Wirksame Länge [cm]" <- w94
        "Primärwindungszahl" <- w65
        "Sekundärwindungszahl" <- w93
        "Messwiderstand [Ohm]" <- w83
        "Spannungsteilerverhältnis (1/x)" <- w92
        n31 = invoke on="Hystereseschleife und Kom.Kurve / Preview" class="XYGraph (strict)" method="Reinit To Default"(error in=w101) -> ()  [unwired: 2 in, 3 out]
        n32 = Divide(x=w93, y=w92) -> (x/y=w77:dbl)
        "TP" <- w77
        n33 = Multiply(x=100.0, y=w65) -> (x*y=w97:dbl)
        n34 = Multiply(x=w94, y=w83) -> (x*y=w96:dbl)
        n35 = Multiply(x=w95, y=w77) -> (x*y=w99:dbl)
        n36 = Divide(x=w97, y=w96) -> (x/y=w75:dbl)
        "Faktor2" <- w75
        n37 = Divide(x=1000000.0, y=w99) -> (x/y=w76:dbl)
        "Faktor1" <- w76
        n38 = Bundle By Name(cluster=w84, "Messung Neukurve.H - Neukurve Array"=w66, "Messung Neukurve.B - Neukurve Array"=w66, "GUI Einstellungen.Minimale Spannung FG"="Minimale Spannung [V]", "Messung Neukurve.Anzahl Messpunkte Neukurve"="Anz. Messpunkte Kommutierungskurve", "Messung Neukurve.Neukurve Messen?"="Kommutierungskurve messen?", "GUI Daten"="GUI Parameter", "GUI Einstellungen.Anzahl der Messpunkte"="Anzahl der Oszi-Messpunkte", "GUI Einstellungen.VISA Name Oszilloscope"="VISA Name Oszilloscope", "GUI Einstellungen.Maximale Spannung FG"="Maximale Spannung [V]", "GUI Einstellungen.VISA Name Frequenzgenerator"="VISA Name Frequenzgen.", "GUI Einstellungen.Faktor1"=w76, "GUI Einstellungen.Faktor2"=w75, "GUI Einstellungen.Theoretische Primärwindungszahl"=w77, "GUI Einstellungen.Maximal Strom [A]"="Maximal zulässiger Strom [A]") -> (w85:T3)
        n39 = local write "Status"(TRUE ("Status")) -> ()
      }
      frame "Initialisieren Hardware" {
        n40 = Format Into String(w108) -> (resulting string=w109:string)  [unwired: 3 in, 1 out]
        n41 = local write "Aktueller Zustand"(w109) -> ()
        n42 = Unbundle By Name(w115) -> ("GUI Einstellungen.VISA Name Oszilloscope"=w112:refnum<visa-resource-name>, "GUI Einstellungen.VISA Name Frequenzgenerator"=w111:refnum<visa-resource-name>)
        n43 = call "FrequenzgeneratorInit.vi"("Error_in"=w114, "VISA Name FG in(FG)"=w111) -> ("Error_out"=w113:errorcluster)  [unwired: 9 in]
        n44 = call "OszilloscopeInit.vi"("Error_in"=w113, "VISA Name OZ in(OZ)"=w112) -> ("Error_out"=w107:errorcluster)  [unwired: 9 in]
        n45 = call <vilib>:"General Error Handler.vi"("error in (no error)"=w107) -> ("error?"=w103:bool)  [unwired: 10 in, 4 out]
        n46 = local write "Status"(TRUE ("Status")) -> ()
        n47 = Select(t=State."Warten auf Event" ("Next State"), s=w103, f=State."Flussdichte Einstellen" ("Next State")) -> (s? t:f=w106:T4)
      }
      frame "Flussdichte Einstellen" {
        n48 = Format Into String(w129) -> (resulting string=w130:string)  [unwired: 3 in, 1 out]
        n49 = local write "Aktueller Zustand"(w130) -> ()
        n50 = Unbundle By Name(w127) -> ("GUI Einstellungen"=w126:T5, "GUI Daten"=w134:T6, "Globale Variablen"=w124:T7)
        n51 = call "FlussdichteAnpassen.vi"("Error in"=w133, "Globale Variablen"=w124, "GUI Data"=w134, "GUI Einstellungen"=w126) -> ("Error out"=w128:errorcluster, "Globale Variablen out"=w123:T8, "GUI Data out"=w132:T6, "GUI Einstellungen out"=w125:T5)  [unwired: 4 in]
        n52 = Bundle By Name(cluster=w127, "GUI Einstellungen"=w125, "GUI Daten"=w132, "Globale Variablen"=w123) -> (w116:T3)
        n53 = Unbundle By Name(w116) -> ("Globale Variablen.Strombegrenzung aktiv?"=w119:bool, "Globale Variablen.Abbruch Messung"=w120:bool)
        n54 = Or(x=w119, y=w120) -> (x .or. y?=w118:bool)
        n55 = local write "Status"(TRUE ("Status")) -> ()
        n56 = Select(t=State."Entmagnetisieren 2" ("Next  State"), s=w118, f=State."Chk Flussdichte Anpassung" ("Next  State")) -> (s? t:f=w117:T4)
      }
      frame "Chk Flussdichte Anpassung" {
        n57 = Format Into String(w141) -> (resulting string=w142:string)  [unwired: 3 in, 1 out]
        n58 = local write "Aktueller Zustand"(w142) -> ()
        n59 = Unbundle By Name(w146) -> ("GUI Einstellungen"=w137:T5, "Globale Variablen"=w139:T7)
        n60 = call "Anpassungspruefung.vi"("Error in"=w144, "Globale Variablen"=w139, "GUI Einstellungen"=w137) -> ("Error out"=w145:errorcluster, "Globale Variablen out"=w138:T8, "GUI Einstellungen out"=w136:T5)  [unwired: 6 in]
        n61 = Bundle By Name(cluster=w146, "GUI Einstellungen"=w136, "Globale Variablen"=w138) -> (w140:T3)
        n62 = local write "Status"(TRUE ("Status")) -> ()
      }
      frame "Messung Hystereseschleife" {
        n63 = Format Into String(w155) -> (resulting string=w156:string)  [unwired: 3 in, 1 out]
        n64 = local write "Aktueller Zustand"(w156) -> ()
        n65 = Unbundle By Name(w159) -> ("Messung Hystereseschleife"=w154:T9, "GUI Einstellungen"=w153:T5, "GUI Daten"=w152:T6, "Globale Variablen"=w148:T7)
        n66 = call "MessungHystereseschleife.vi"("Messung Hystereseschleife"=w154, "Error in"=w158, "Globale Variablen"=w148, "GUI Data"=w152, "GUI Einstellungen"=w153) -> ("Error out"=w160:errorcluster, "Globale Variablen out"=w147:T8, "GUI Data out"=w151:T6, "GUI Einstellungen out"=w150:T5, "Messung Hystereseschleife out"=w149:T9)  [unwired: 2 in]
        n67 = Bundle By Name(cluster=w159, "Messung Hystereseschleife"=w149, "GUI Einstellungen"=w150, "GUI Daten"=w151, "Globale Variablen"=w147) -> (w162:T3)
        n68 = local write "Status"(TRUE ("Status")) -> ()
      }
      frame "Entmagnetisieren" {
        n69 = Format Into String(w164) -> (resulting string=w165:string)  [unwired: 3 in, 1 out]
        n70 = local write "Aktueller Zustand"(w165) -> ()
        n71 = Unbundle By Name(w176) -> ("GUI Einstellungen.Minimale Spannung FG"=w166:dbl, "GUI Daten.Frequenz [Hz]"=w174:dbl, "GUI Einstellungen.VISA Name Frequenzgenerator"=w173:refnum<visa-resource-name>, "Globale Variablen.Spannungsabweichung"=w172:dbl)
        n72 = call "Entmagnetisierung.vi"("minimale Spannung FG"=w166, "Frequenz"=w174, "error in (no error)"=w175, "Spannungsabweichung"=w172, "VISA Name FG in"=w173) -> ("error out"=w167:errorcluster)  [unwired: 5 in, 1 out]
        n73 = local read "Kommutierungskurve messen?"() -> (w170:bool)
        n74 = local write "Status"(TRUE ("Status")) -> ()
        n75 = Select(t=State."Messung Kommutierungskurve" ("(Value Not Used)"), s=w170, f=State."Ausgabe Diagramm" ("(Value Not Used)")) -> (s? t:f=w169:T4)
      }
      frame "Messung Kommutierungskurve" {
        n76 = Format Into String(w178) -> (resulting string=w179:string)  [unwired: 3 in, 1 out]
        n77 = local write "Aktueller Zustand"(w179) -> ()
        n78 = Unbundle By Name(w186) -> ("GUI Einstellungen.Minimale Spannung FG"=w180:dbl, "Messung Neukurve.Anzahl Messpunkte Neukurve"=w182:i8, "GUI Einstellungen.Faktor1"=w183:dbl, "GUI Einstellungen.Faktor2"=w184:dbl, "Globale Variablen.Spannungsabweichung"=w189:dbl, "GUI Einstellungen.Maximale Spannung FG"=w188:dbl, "GUI Daten.Frequenz [Hz]"=w191:dbl, "GUI Einstellungen.Anzahl der Messpunkte"=w192:i32, "GUI Einstellungen.VISA Name Oszilloscope"=w193:refnum<visa-resource-name>, "GUI Einstellungen.VISA Name Frequenzgenerator"=w194:refnum<visa-resource-name>)
        n79 = call "MessungNeukurve.vi"("Spannungs Abweichung"=w189, "maximale Spannung FG"=w188, "Frequenz (1000 Hz)"=w191, "Messpunkte Oszi (6000)"=w192, "VISA Name OZ In (OZ)"=w193, "VISA Name FG in"=w194, "error in"=w196, "Faktor 2"=w184, "Faktor 1"=w183, "Anzahl Messpunkte Neukurve"=w182, "minimale Spannung FG"=w180) -> ("Output B Array"=w185:dbl[], "Output H Array"=w187:dbl[], "error out"=w195:errorcluster)  [unwired: 12 in, 2 out]
        n80 = Bundle By Name(cluster=w186, "Messung Neukurve.B - Neukurve Array"=w185, "Messung Neukurve.H - Neukurve Array"=w187) -> (w190:T3)
        n81 = local write "Status"(TRUE ("Status")) -> ()
      }
      frame "Entmagnetisieren 2" {
        n82 = Format Into String(w205) -> (resulting string=w204:string)  [unwired: 3 in, 1 out]
        n83 = local write "Aktueller Zustand"(w204) -> ()
        n84 = Unbundle By Name(w198) -> ("GUI Einstellungen.Minimale Spannung FG"=w206:dbl, "GUI Daten.Frequenz [Hz]"=w210:dbl, "GUI Einstellungen.VISA Name Frequenzgenerator"=w211:refnum<visa-resource-name>, "Globale Variablen.Spannungsabweichung"=w212:dbl)
        n85 = call "Entmagnetisierung.vi"("minimale Spannung FG"=w206, "Frequenz"=w210, "error in (no error)"=w209, "Spannungsabweichung"=w212, "VISA Name FG in"=w211) -> ("error out"=w208:errorcluster)  [unwired: 5 in, 1 out]
        n86 = Unbundle By Name(w198) -> ("Globale Variablen.Strombegrenzung aktiv?"=w199:bool, "Globale Variablen.Abbruch Messung"=w200:bool)
        n87 = Or(x=w199, y=w200) -> (x .or. y?=w197:bool)
        n88 = local write "Status"(TRUE ("Status")) -> ()
        n89 = Select(t=State."Ende" ("Next  State"), s=w197, f=State."Ausgabe Diagramm" ("Next  State")) -> (s? t:f=w201:T4)
      }
      frame "Ausgabe Diagramm" {
        w230 = State."Ende"  # Nächster Zustand
        n90 = Format Into String(w220) -> (resulting string=w219:string)  [unwired: 3 in, 1 out]
        n91 = local write "Aktueller Zustand"(w219) -> ()
        n92 = Unbundle By Name(w225) -> ("Messung Hystereseschleife.H - Hysterese Array"=w218:dbl[], "Messung Hystereseschleife.B - Hysterese Array"=w217:dbl[])
        n93 = Unbundle By Name(w225) -> ("Messung Neukurve.H - Neukurve Array"=w228:dbl[], "Messung Neukurve.B - Neukurve Array"=w227:dbl[], "Messung Hystereseschleife.Hystereseverluste"=→"Hystereseverluste [W]":dbl, "Messung Hystereseschleife.Remanenz"=→"Remanenz [T]":dbl, "Messung Hystereseschleife.Koerzitivfeldstärke"=→"Koerzitivfeldstärke [A/m]":dbl, "Messung Hystereseschleife.Hmax"=→"Hmax [A/m]":dbl, "Messung Hystereseschleife.Bmax"=→"Bmax [T]":dbl)
        n94 = Bundle("H - Hysterese Array"=w218, "B - Hysterese Array"=w217) -> (w224:T10)  [unwired: 1 in]
        n95 = Bundle("H - Neukurve Array"=w228, "B - Neukurve Array"=w227) -> (w226:T11)  [unwired: 1 in]
        n96 = Build Array(w224, w226) -> (→"Hystereseschleife und Kom.Kurve" →"Hystereseschleife und Kom.Kurve / Preview":T12)
        n97 = Get Date/Time In Seconds() -> (seconds since 1Jan1904=→"Datum/Uhrzeit":timestamp)
        n98 = local write "Status"(TRUE ("Status")) -> ()
      }
      frame "Ende" {
        n99 = local write "Aktueller Zustand"("" ("Aktueller Zustand")) -> ()
        n100 = Unbundle By Name(w241) -> ("GUI Einstellungen.VISA Name Frequenzgenerator"=w235:refnum<visa-resource-name>, "GUI Einstellungen.VISA Name Oszilloscope"=w236:refnum<visa-resource-name>)
        n101 = call "AnsteuerungOszilloscope.vi"("Error_in"=w242, "Eingangs-String"=":SYStEM:LOCK OFF;", "VISA Name OZ in(OZ)"=w236) -> ("Error_out"=w237:errorcluster)  [unwired: 6 in, 2 out]
        n102 = call "AnsteuerungFrequenzgenerator.vi"("Error_in"=w237, "Eingangs-String"=":OUTP OFF;" ("true string"), "VISA Name FZ in(FZ)"=w235) -> ("Error_out"=w232:errorcluster)  [unwired: 5 in, 2 out]
        n103 = local write "Status"(FALSE ("Status")) -> ()
      }
      frame "Plot aufnehmen" {
        n104 = invoke on="Hystereseschleife und Kom.Kurve" class="XYGraph (strict)" method="Get Image"(error in=w247) -> (error out=w246:errorcluster, "image data"=w248:T13)  [unwired: 5 in, 4 out]
        n105 = call <vilib>:"Write PNG File.vi"("error in (no error)"=w246, "image data"=w248) -> ("error out"=w245:errorcluster)  [unwired: 8 in, 1 out]
        n106 = call <vilib>:"General Error Handler.vi"("error in (no error)"=w245) -> ()  [unwired: 10 in, 5 out]
        n107 = local write "Status"(FALSE ("Status")) -> ()
      }
      frame "Ansicht speichern" {
        n108 = invoke on="Tab Control" class="TabCtl (strict)" method="Get Image"(error in=w252) -> (error out=w255:errorcluster, "image data"=w254:T13)  [unwired: 5 in, 4 out]
        n109 = call <vilib>:"Write PNG File.vi"("error in (no error)"=w255, "image data"=w254) -> ("error out"=w253:errorcluster)  [unwired: 8 in, 1 out]
        n110 = call <vilib>:"General Error Handler.vi"("error in (no error)"=w253) -> ()  [unwired: 10 in, 5 out]
        n111 = local write "Status"(FALSE ("Status")) -> ()
      }
      frame "Excel Export" {
        n112 = invoke on="Hystereseschleife und Kom.Kurve" class="XYGraph (strikt)" method="Export Plot Data To Excel"(error in=w260, "Plot"=1) -> (error out=w257:errorcluster)  [unwired: 2 in, 3 out]
        n113 = call <vilib>:"General Error Handler.vi"("error in (no error)"=w257) -> ()  [unwired: 10 in, 5 out]
        n114 = local write "Status"(FALSE ("Status")) -> ()
      }
    }
    n115 = Or(x=w7, y=w6) -> (x .or. y?=w8:bool)
  }
  n116 = call <vilib>:"General Error Handler.vi"("error in (no error)"=w3) -> ("error out"=w2:errorcluster)  [unwired: 10 in, 4 out]
  n117 = disable-structure shown="RUN_TIME_ENGINE==True" {
    disable-tunnel: w2 -> [_ w263]
    frame condition #0 (active) {
    }
    frame condition #1 {
      # "Call Quit LabVIEW\nif running as a\nbuilt application."
      n118 = Quit LabVIEW(quit? (T)=w263) -> ()
    }
  }
